vi "niFpgaIPINodeGlobal.vi"() -> ()   [LabVIEW 2017]
panel:
  in  "OFFSET SIM":u32=7
  in  "OFFSET SYN":u32=21
  in  "OFFSET SIM DLG":u32=49
  out "CONTRACTED VIEW":picture
  out "EXCLAMATATION":picture
  in  "OVERCLOCK ID":string="ni_overclock_unique_id"
  out "LOGO":picture
  in  "CONFIG PAGE6 ID":string="IPIN_MENU_CONFIG_PAGE6"
  in  "CONFIG PAGE5 ID":string="IPIN_MENU_CONFIG_PAGE5"
  in  "CONFIG PAGE4 ID":string="IPIN_MENU_CONFIG_PAGE4"
  in  "CONFIG PAGE3 ID":string="IPIN_MENU_CONFIG_PAGE3"
  in  "CONFIG PAGE2 ID":string="IPIN_MENU_CONFIG_PAGE2"
  in  "CONFIG PAGE1 ID":string="IPIN_MENU_CONFIG_PAGE1"
  in  "CONFIG MENU ID":string="IPIN_MENU_CONFIG"
  in  "SMALL ICON MENU ID":string="IPIN_MENU_SMALL_ICON"
  in  "BIG ICON MENU ID":string="IPIN_MENU_BIG_ICON"
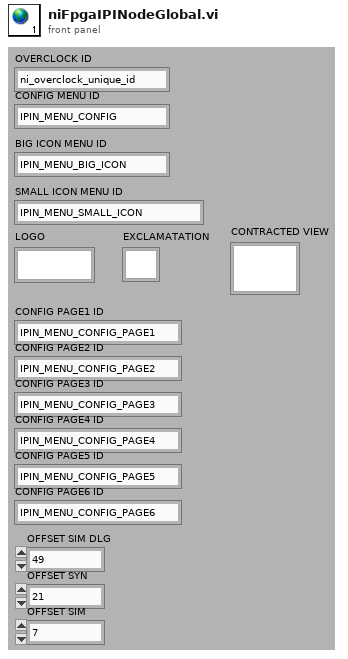
[diagram p1: front panel]
diagram:
